vi "ChannelType_1D-Array-CSG.vi"(9 "error in":errorcluster, 11 "Array in":csg[](array[numeric])) -> (1 "error out":errorcluster, 2 "ChannelType":sgl, 3 "Array out":csg[](array[numeric]))   [LabVIEW 2020, in "OpenLvVision_OpenCv.lvlib"]
uses:
  OpenLvVision_OpenCv.lvlib
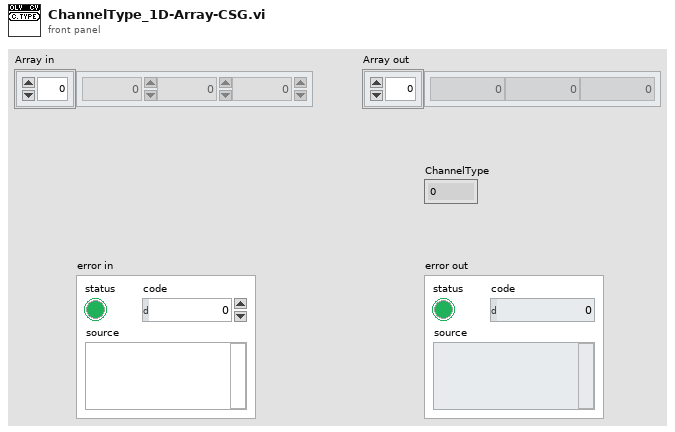
[diagram p1: front panel]
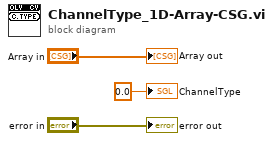
[diagram p0: block diagram]
diagram:
  "error out" <- "error in"
  "Array out" <- "Array in"
  "ChannelType" <- sgl 0.0
